vi "Measurement Logic.vi"(8 "error in":errorcluster, 9 "measurement configuration":T2={"Input Terminal Name"="Lorem ipsum dolor sit", "Counter Interface"="", "Active Edge"=10171, "Pulses"=0, "Timeout (s)"=0} {"Active Edge" items=["Rising"=10280, "Falling"=10171]}, 10 "measure call context in":refnum<class "Measure Call Context.lvclass">) -> (0 "error out":errorcluster, 1 "Measurements Resuts":T1, 2 "measure call context out":refnum<class "Measure Call Context.lvclass">)   [LabVIEW 2025, in "Count Edges.lvclass"]
doc: "Contains the core logic for executing the measurement."
uses:
  Count Edges.lvclass
  <vilib>/Plug-In SDKs/Measurements/Measure Call Context/Measure Call Context.lvclass
  Measurement Configuration.ctl
  Measurement Results.ctl
  <vilib>/DAQmx/read.llb/DAQmx Read (Counter U32 1Chan 1Samp).vi
  <vilib>/DAQmx/create/channels.llb/DAQmx Create Channel (CI-Count Edges).vi
  <vilib>/DAQmx/miscellaneous.llb/DAQmx Fill In Error Info.vi
  <extravilib>/ChannelInstances/Event Messenger-bool/Instantiate.vi
  Count Edges.lvclass/Count Edges.ctl
  <resource>/objmgr/daqmx.rc
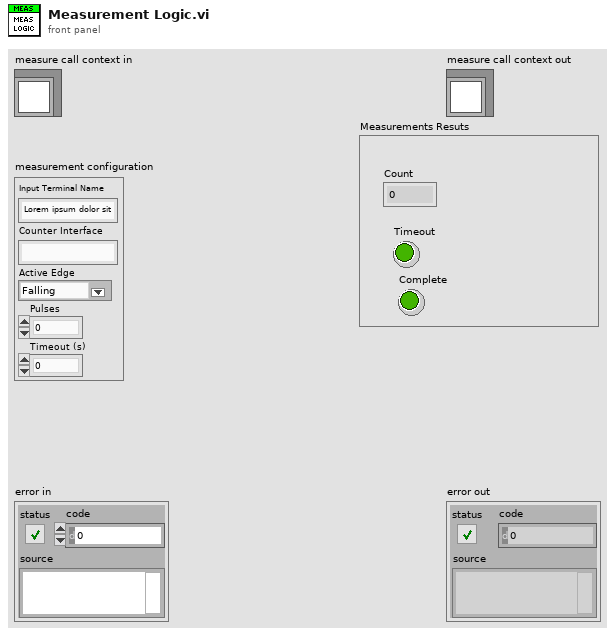
[diagram p1: front panel]
types:
  T1 = typedef "Count Edges.lvclass/Measurement Results.ctl" = cluster{"Count":u32, "Timeout":bool, "Complete":bool}
  T2 = typedef "Count Edges.lvclass/Measurement Configuration.ctl" = cluster{"Input Terminal Name":string, "Counter Interface":string, "Active Edge":i32, "Pulses":u32, "Timeout (s)":u32}
  T3 = typedef "Event Messenger-bool.lvlib/))Channel.ctl" = refnum<queue>
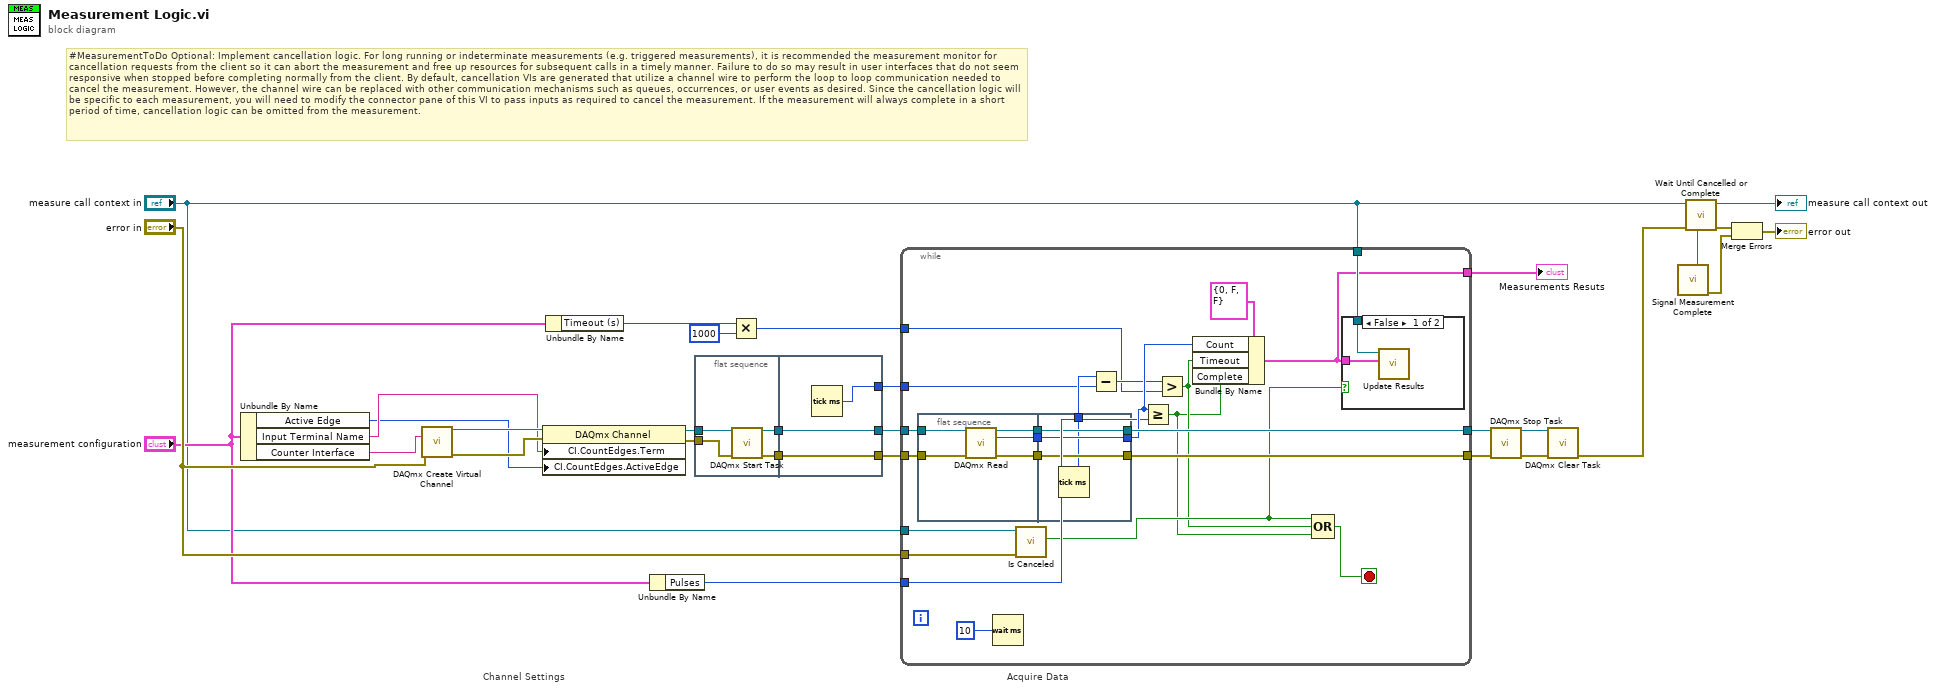
[diagram p0: block diagram]
diagram:
  # "Acquire Data"
  # "Channel Settings"
  # "#MeasurementToDo Optional: Implement cancellation logic. For long running or indeterminate measurements (e.g. triggered measurements), it is recommended the measurement monitor for cancellation requests from the client so it can abort the measurement and free up resources for subsequent calls in a timely manner. Failure to do so may result in user interfaces that do not seem responsive when stopped before completing normally from the client. By default, cancellation VIs are generated that utilize a channel wire to perform the loop to loop communication needed to cancel the measurement. However, the channel wire can be replaced with other communication mechanisms such as queues, occurrences, or user events as desired. Since the cancellation logic will be specific to each measurement, you will need to modify the connector pane of this VI to pass inputs as required to cancel the measurement. If the measurement will always complete in a short period of time, cancellation logic can be omitted from the measurement."
  n1 = Unbundle By Name("measurement configuration") -> ("Active Edge"=w14:i32, "Input Terminal Name"=w15:string, "Counter Interface"=w16:string)
  n2 = call-poly <vilib>:"DAQmx Create Virtual Channel.vi"("counter"=w16, "error in"="error in") -> ("task out"=w22:refnum<k21>, "error out"=w21:errorcluster)  [unwired: 12 in]
  n3 = property class="DAQmx Channel"(reference=w22, error in=w21, "CI.CountEdges.Term"=w15, "CI.CountEdges.ActiveEdge"=w14) -> (reference out=w3:refnum<k21>, error out=w24:errorcluster)
  n4 = Unbundle By Name("measurement configuration") -> ("Timeout (s)"=w9:u32)
  n5 = Unbundle By Name("measurement configuration") -> ("Pulses"=w12:u32)
  n6 = flat-sequence {
    tunnel: w24 -> [w34]
    tunnel: [w33] -> w7
    tunnel: [w32] -> w6
    tunnel: w3 -> [w31]
    tunnel: [w37] -> w23
    tunnel: w7 -> [w36]
    tunnel: w6 -> [w37]
    tunnel: [w36] -> w5
    tunnel: [w35] -> w4
    frame #0 {
      n7 = call <vilib>:"DAQmx Start Task.vi"("task/channels in"=w31, "error in"=w34) -> ("task out"=w33:refnum<k21>, "error out"=w32:errorcluster)  [unwired: 12 in]
    }
    frame #1 {
      n8 = Tick Count (ms)() -> (millisecond timer value=w35:u32)
    }
  }
  n9 = Multiply(x=w9, y=u32 1000) -> (x*y=w8:u32)
  n10 = while {
    tunnel: w23 -> [w60]
    tunnel: [w58] -> w19
    tunnel: [w59] -> w20
    tunnel: "error in" -> [w56]
    tunnel: "measure call context in" -> [w55]
    tunnel: w12 -> [w53]
    tunnel: w4 -> [w48]
    tunnel: w8 -> [w46]
    tunnel: w5 -> [w45]
    tunnel: "measure call context in" -> [w43]
    tunnel: [w42] -> w1
    stop <- w41 stop-if-true
    n11 = flat-sequence {
      tunnel: w60 -> [w67]
      tunnel: [w66] -> w52
      tunnel: [w65] -> w51
      tunnel: [w64] -> w50
      tunnel: w45 -> [w63]
      tunnel: [w69] -> w54
      tunnel: [w70] -> w58
      tunnel: [w71] -> w59
      tunnel: w52 -> [w71]
      tunnel: w51 -> [w70]
      tunnel: w50 -> [w69]
      tunnel: [w68] -> w49
      frame #0 {
        n12 = call-poly <vilib>:"DAQmx Read.vi"("task/channels in"=w63, "error in"=w67) -> ("task out"=w66:refnum<k21>, "data"=w64:u32, "error out"=w65:errorcluster)  [unwired: 11 in]
      }
      frame #1 {
        n13 = Tick Count (ms)() -> (millisecond timer value=w68:u32)
      }
    }
    n14 = Wait (ms)(milliseconds to wait=u32 10 ("Loop Time (ms)")) -> ()  [unwired: 1 out]
    n15 = call <vilib>:"Is Canceled.vi"("error in"=w56, "measure call context in"=w55) -> ("is canceled?"=w40:bool)  [unwired: 7 in, 2 out]
    n16 = Subtract(x=w49, y=w48) -> (x-y=w47:u32)
    n17 = Greater Or Equal?(x=w54, y=w53) -> (x >= y?=w38:bool)
    n18 = Greater?(x=w47, y=w46) -> (0:w39:bool)
    n19 = Bundle By Name(cluster=T1 {"Count"=0, "Timeout"=FALSE, "Complete"=FALSE} ("measurement results"), "Count"=w54, "Timeout"=w39, "Complete"=w38) -> (w42:T1)
    n20 = Compound Arithmetic op=OR(w40, w39, w38) -> (w41:bool)
    n21 = case shown="False" w40 {
      tunnel: w42 -> [w62 _]
      tunnel: w43 -> [w61 _]
      frame False {
        n22 = call <vilib>:"Update Results.vi"("measurement results"=w62, "measure call context in"=w61) -> ()  [unwired: 8 in, 2 out]
      }
      frame True {
      }
    }
  }
  "Measurements Resuts" <- w1
  n23 = call <vilib>:"DAQmx Stop Task.vi"("task/channels in"=w20, "error in"=w19) -> ("task out"=w17:refnum<k21>, "error out"=w18:errorcluster)  [unwired: 12 in]
  n24 = call <vilib>:"DAQmx Clear Task.vi"("task in"=w17, "error in"=w18) -> ("error out"=w13:errorcluster)  [unwired: 13 in]
  n25 = call "Signal Measurement Complete.vi"() -> ("error out"=w27:errorcluster, "done channel"=w28:T3)  [unwired: 10 in]
  n26 = call "Wait Until Cancelled or Complete.vi"("done channel"=w28, "error in (no error)"=w13, "measure call context in"="measure call context in") -> ("error out"=w26:errorcluster, "measure call context out"=→"measure call context out":refnum<class "Measure Call Context.lvclass">)  [unwired: 7 in]
  n27 = Merge Errors(w26, w27) -> (→"error out":errorcluster)
